vi "Get Buttons Values.vi"(8 "error in (no error)":errorcluster, 11 "GripsMaster in":refnum<class "GripsMaster.lvclass">) -> (0 "error out":errorcluster, 2 "Grips Buttons":T1, 3 "GripsMaster out":refnum<class "GripsMaster.lvclass">)   [LabVIEW 2013, in "GripsMaster.lvclass"]
uses:
  GripsMaster.lvclass
  controls/Grips Buttons.ctl
  GripsMaster.lvclass/GripsMaster.ctl
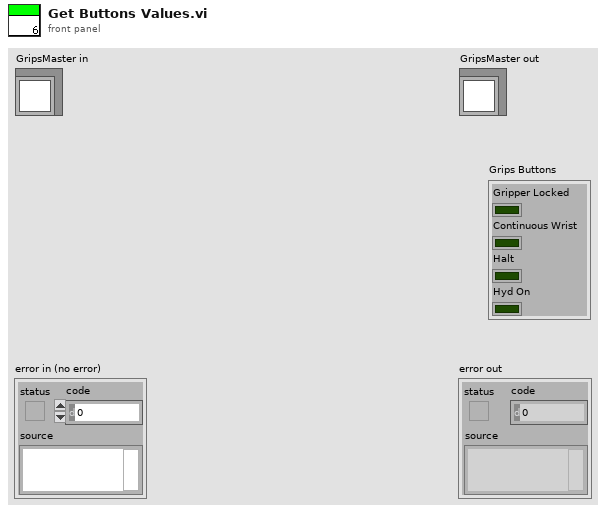
[diagram p1: front panel]
types:
  T1 = typedef "Grips Buttons.ctl" = cluster{"Gripper Locked":bool, "Continuous Wrist":bool, "Halt":bool, "Hyd On":bool}
  T2 = typedef "Digital Values.ctl" = cluster{"names":string[], "values":bool[]}
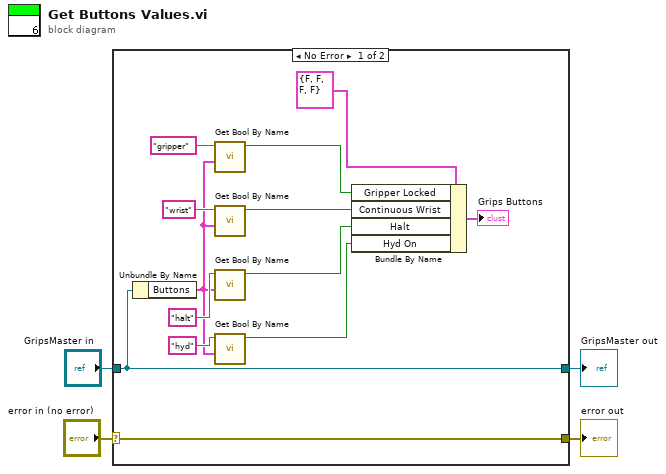
[diagram p0: block diagram]
diagram:
  n1 = case shown="No Error" "error in (no error)" {
    selector: "error in (no error)" -> [w17 w19]
    tunnel: [w17 w19] -> w3
    tunnel: [w14 w18] -> w1
    tunnel: "GripsMaster in" -> [w14 w18]
    frame No Error {
      n2 = Unbundle By Name(w14) -> ("Buttons"=w7:T2)
      n3 = call "Get Bool By Name.vi"("name"="gripper", "Digital Values"=w7) -> ("result"=w12:bool)  [unwired: 7 in, 1 out]
      n4 = call "Get Bool By Name.vi"("name"="wrist", "Digital Values"=w7) -> ("result"=w10:bool)  [unwired: 7 in, 1 out]
      n5 = call "Get Bool By Name.vi"("name"="halt", "Digital Values"=w7) -> ("result"=w6:bool)  [unwired: 7 in, 1 out]
      n6 = call "Get Bool By Name.vi"("name"="hyd", "Digital Values"=w7) -> ("result"=w5:bool)  [unwired: 7 in, 1 out]
      n7 = Bundle By Name(cluster=T1 {"Gripper Locked"=FALSE, "Continuous Wrist"=FALSE, "Halt"=FALSE, "Hyd On"=FALSE} ("Grips Buttons"), "Gripper Locked"=w12, "Continuous Wrist"=w10, "Halt"=w6, "Hyd On"=w5) -> (→"Grips Buttons":T1)
    }
    frame Error {
    }
  }
  "error out" <- w3
  "GripsMaster out" <- w1
